vi "OBD_speed.vi"(7 "error in":errorcluster, 9 "OBD VISA Refnum":refnum<visa-resource-name>) -> (0 "error out":errorcluster, 1 "Speed (km/h)":u32, 2 "OBD VISA Out":refnum<visa-resource-name>)   [LabVIEW 2020]
doc: "The Advanced Serial Read and Write example performs a Serial Port Read, a Serial Port Write, or a combination of these actions while setting some advanced serial features like buffer size, termination characters, and XON/XOFF flow control. The user selects the actions (read or write) on the front panel. If both are selected, the VI will write the data first, read the data and then close the VISA session that is opened to the port. \n\nThe parameters set for the serial port must match the parameters of the connected instrument or device. In this example, the bytes to read parameter specifies the number of bytes that the serial port reads. If there were more bytes at the port than the number specified in bytes to read, those bytes would not be read. Also, if you specify to read more bytes than the number of bytes actually read, you might receive a timeout error message.\n\nINSTRUCTIONS:\n1) Select the serial resource and configuration parameters (baud rate, data bits, parity, stop bits, flow control).\n2) Termination character can be enabled and set. Also, set the required input buffer size prior to running the example.\n3) Select the operations to be performed. \n4) Connect the serial port to your device. If no device is available, perform a loopback test by doing one of the following. Short pins 2 and 3 on a RS-232 cable or short pin 4 to pin 8 and pin 5 to pin 9 on a RS-485/422 cable. \n5) Run the VI to see the data read. (The \"read string\" will match the \"string to write\" if a loopback test was performed.)\n\nThis example exposes several advanced features that you may need for your application. Not all applications need all the features shown in this example. The input buffer size is likely an important setting that you want to control in your application. This example expands upon the flow control option for XON and XOFF, allowing the user to choose those control characters. The timeout parameter has been brought to the front panel so a user can specify the time period the VISA Read will wait for the number of bytes to read before timing out. Also, the user has several controls for the termination character, which is discussed later.\n\nNote that you can press the write and read buttons and change the bytes to read parameters on the fly, while the example is running. However, you must stop the example to change the other configuration parameters after the example has started running, and then run again.\n\nSet the I/O buffer size slightly higher the amount of data you expect to receive. This is very important for applications that don't use flow control, as you may lose characters if the receive buffer overflows.\n\nSetting the timeout period ensures that the operation returns with a timeout error if the operation cannot be performed in the specified time period. \n\nSome devices require a termination character in order to identify the end of command strings. Some devices send a termination character to signify the end of data to be read. \n\nThis example shows how you can end the Read operation once a termination character is detected in the buffer and/or append a termination character at the end of the Write data. To enable the Read to end on a termination character, use the VISA Configure Serial Port or use the VISA Properties Serial End Mode for Reads, Termination Character Enable, and Termination Character. To end the Write with a termination character, use the VISA Properties Serial End Mode for Writes, the Send End Enable, and Termination Character. In this example, the same termination character is used for both the Read and the Write. You can specify two different characters for your application, if desired.\n\nYour application may require specific characters for the XON/XOFF Flow Control. You can specify these characters with the VISA Properties Flow Control XOFF Character and Flow Control XON Character. Note that if the standard XON and XOFF characters are used, then decimal 17 and 19 are unavailable for data values. Remember that using flow control and setting an adequate buffer size allow you to prevent buffer overflows."
uses:
  terminal.vi
panel:
  out "Speed (km/h)":u32(graph)
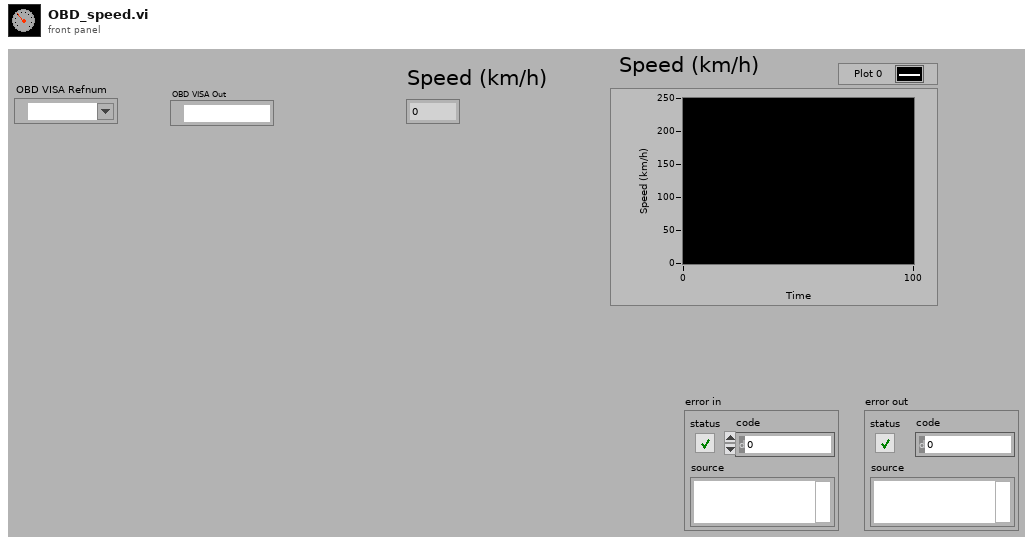
[diagram p1: front panel]
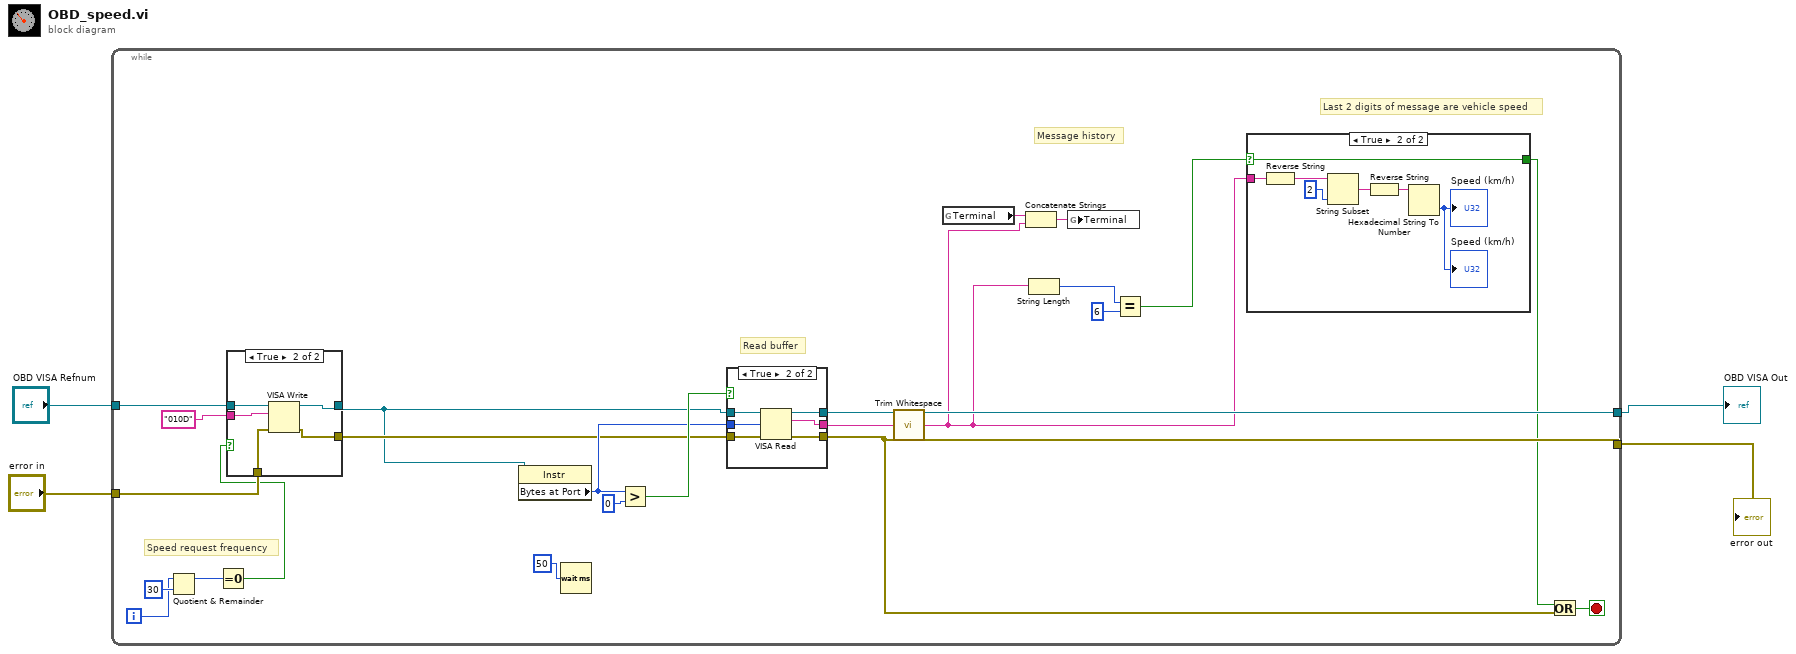
[diagram p0: block diagram]
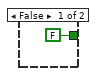
[diagram p3: hidden frame]
diagram:
  n1 = while {
    tunnel: [w26] -> w1
    tunnel: [w17] -> w4
    tunnel: "error in" -> [w15]
    tunnel: "OBD VISA Refnum" -> [w14]
    i -> [w8]
    stop <- w22 stop-if-true
    # "Speed request frequency"
    # "Read buffer"
    # "Last 2 digits of message are vehicle speed"
    # "Message history"
    n2 = Quotient & Remainder(x=w8, y=30) -> (x-y*floor(x/y)=w9:i32)  [unwired: 1 out]
    n3 = Equal To 0?(x=w9) -> (x = 0?=w7:bool)
    n4 = case shown="True" w7 {
      tunnel: w15 -> [w29 w35]
      tunnel: w14 -> [w30 w34]
      tunnel: [w29 w33] -> w13
      tunnel: "010D" ("String") -> [_ w32]
      tunnel: [w30 w31] -> w11
      frame False {
      }
      frame True {
        n5 = VISA Write(VISA resource name=w34, write buffer=w32, error in (no error)=w35) -> (VISA resource name out=w31:refnum<visa-resource-name>, error out=w33:errorcluster)  [unwired: 1 out]
      }
    }
    n6 = property class="Instr"(reference=w11) -> ("Bytes at Port"=w25:u32)  [unwired: 1 in, 2 out]
    n7 = Wait (ms)(milliseconds to wait=u32 50) -> ()  [unwired: 1 out]
    n8 = Greater?(x=w25, y=u32 0) -> (0:w27:bool)
    n9 = case shown="True" w27 {
      tunnel: [w44 w51] -> w17
      tunnel: [w45 w50] -> w26
      tunnel: w13 -> [w44 w49]
      tunnel: w11 -> [w45 w48]
      tunnel: [_ w47] -> w24
      tunnel: w25 -> [_ w46]
      frame False {
      }
      frame True {
        n10 = VISA Read(VISA resource name=w48, byte count=w46, error in (no error)=w49) -> (VISA resource name out=w50:refnum<visa-resource-name>, read buffer=w47:string, error out=w51:errorcluster)  [unwired: 1 out]
      }
    }
    n11 = call <vilib>:"Trim Whitespace.vi"("string"=w24) -> ("trimmed string"=w19:string)  [unwired: 1 in]
    n12 = global read "terminal.vi" "Terminal"() -> (w5:string)
    n13 = Concatenate Strings(w5, w19) -> (w23:string)
    n14 = String Length(string=w19) -> (length=w21:i32)
    n15 = global write "terminal.vi" "Terminal"(w23) -> ()
    n16 = Equal?(x=w21, y=6) -> (x = y?=w18:bool)
    n17 = case shown="True" w18 {
      selector: w18 -> [_ w38]
      tunnel: w19 -> [_ w41]
      tunnel: [FALSE w38] -> w16
      frame False {
      }
      frame True {
        n18 = Reverse String(1:w41) -> (0:w43:string)
        n19 = String Subset(string=w43, length (rest)=2 ("length (rest)")) -> (substring=w40:string)  [unwired: 1 in]
        n20 = Reverse String(1:w40) -> (0:w39:string)
        n21 = Hexadecimal String To Number(string=w39) -> (number=→"Speed (km/h)" →"Speed (km/h)":u32)  [unwired: 2 in, 1 out]
      }
    }
    n22 = Or(x=w16, y=w17) -> (x .or. y?=w22:bool)
  }
  "error out" <- w4
  "OBD VISA Out" <- w1
